vi "generator liczb losowych.vi"() -> ()   [LabVIEW 2018]
panel:
  in  "stop":bool
  in  "file path (use dialog)":path
  out "error out":errorcluster
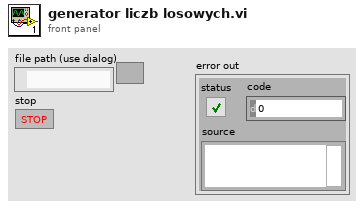
[diagram p1: front panel]
types:
  T1 = enum16{"open", "replace", "create", "open or create", "replace or create", "replace or create with confirmation"}
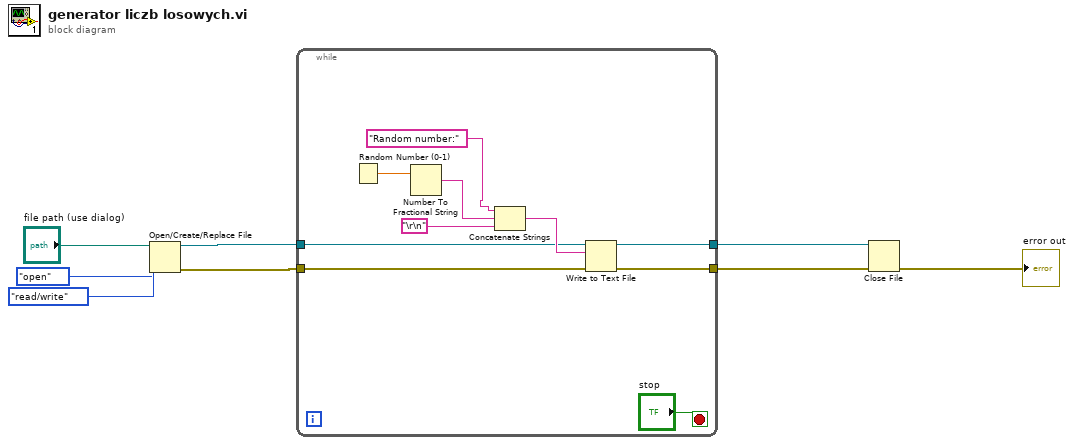
[diagram p0: block diagram]
diagram:
  n1 = Open/Create/Replace File(file path (use dialog)="file path (use dialog)", operation (0:open)=T1."open", access (0:read/write)=enum16{"read/write", "read-only", "write-only"}."read/write") -> (refnum out=w6:refnum<file>, error out=w8:errorcluster)  [unwired: 3 in, 1 out]
  n2 = while {
    tunnel: w8 -> [w13]
    tunnel: [w12] -> w7
    tunnel: w6 -> [w11]
    tunnel: [w10] -> w5
    stop <- "stop" stop-if-true
    n3 = Random Number (0-1)() -> (number: 0 to 1=w14:dbl)
    n4 = Number To Fractional String(number=w14) -> (F-format string=w18:string)  [unwired: 3 in]
    n5 = Concatenate Strings("Random number:", w18, "\r\n") -> (w15:string)
    n6 = Write to Text File(file (use dialog)=w11, text=w15, error in=w13) -> (refnum out=w10:refnum<file>, error out=w12:errorcluster)  [unwired: 1 in, 1 out]
  }
  n7 = Close File(refnum=w5, error in=w7) -> (error out=→"error out":errorcluster)  [unwired: 1 out]
